vi "Set Selection Font by Style.vi"(8 "error in (no error)":errorcluster caption="错误输入（无错误）", 10 "newStyle":i32(ring) items=["Regular"=0, "Bold"=1, "Italic"=2, "Underline"=4, "Strikeout"=8], 11 "RichText 输入":refnum<class "RichText.lvclass"> caption="DNL_LabVIEW Object in") -> (0 "error out":errorcluster caption="错误输出", 3 "RichText 输出":refnum<class "RichText.lvclass"> caption="DNL_LabVIEW Object out")   [LabVIEW 2012, in "RichText.lvclass"]
uses:
  RichText.lvclass
  RichText.lvclass/RichText.ctl
  System.Windows.Forms
  System.Drawing
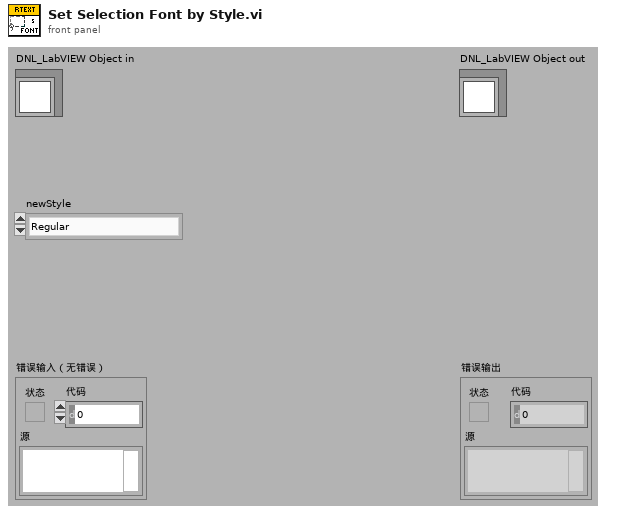
[diagram p1: front panel]
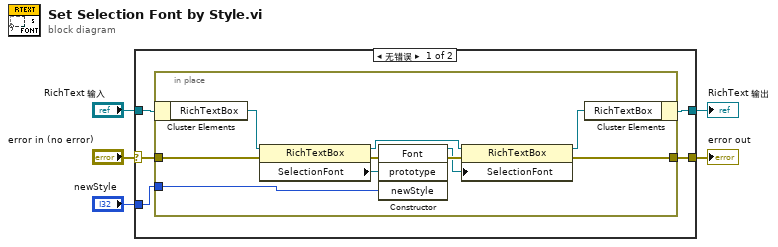
[diagram p0: block diagram]
diagram:
  n1 = case shown="无错误" "error in (no error)" {
    selector: "error in (no error)" -> [w7 w22]
    tunnel: [w6 w22] -> w4
    tunnel: [w9 w21] -> w2
    tunnel: "RichText 输入" -> [w10 w21]
    tunnel: "newStyle" -> [w8 _]
    frame No Error {
      n2 = in-place {
        in-place-border: w8 -> [w16]
        in-place-border: w7 -> [w14]
        in-place-border: [w18] -> w6
        n3 = in-place-cluster #1(w10) -> ("RichTextBox"=w15:refnum<k24>)
        n4 = property class="RichTextBox"(reference=w15, error in=w14) -> (reference out=w11:refnum<k24>, error out=w13:errorcluster, "SelectionFont"=w12:refnum<k24>)
        n5 = constructor class="Font"(error in=w13, "prototype"=w12, "newStyle"=w16) -> (reference out=w17:refnum<k24>, error out=w19:errorcluster)  [unwired: 2 in, 3 out]
        n6 = property class="RichTextBox"(reference=w11, error in=w19, "SelectionFont"=w17) -> (reference out=w20:refnum<k24>, error out=w18:errorcluster)
        n7 = in-place-cluster #1("RichTextBox"=w20) -> (w9:refnum<class "RichText.lvclass">)
      }
    }
    frame Error {
    }
  }
  "error out" <- w4
  "RichText 输出" <- w2
